vi "channel.free.vi"(8 "error in":errorcluster, 11 "Channel in":refnum<class "Channel.lvclass">) -> (0 "error out":errorcluster, 3 "Channel out":refnum<class "Channel.lvclass">)   [LabVIEW 2020, in "Channel.lvclass"]
doc: "Releases the handle and its associated resources."
uses:
  Channel.lvclass
  Channel.lvclass/Channel.ctl
  client.lvlib
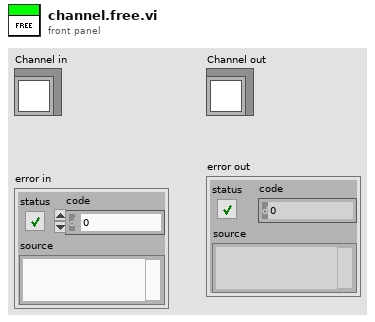
[diagram p1: front panel]
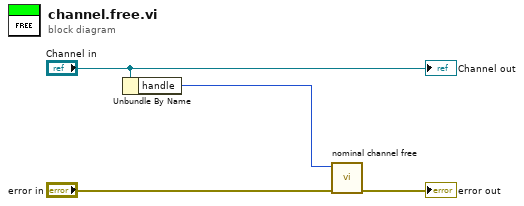
[diagram p0: block diagram]
diagram:
  n1 = Unbundle By Name("Channel in") -> ("handle"=w2:i32)
  n2 = call "nominal channel free.vi"("error in (no error)"="error in", "channel"=w2) -> ("error out"=→"error out":errorcluster)  [unwired: 8 in, 1 out]
  "Channel out" <- "Channel in"
